vi "svc_Complex to Mag2 Spectrum.vi"(4 "complex spectrum":cluster{"f0":dbl, "df":dbl, "spectrum":cdb[]} {"spectrum" format="%.2f"; "df" format="%.2f"; "f0" format="%.2f"}) -> (1 "power spectrum":cluster{"f0":dbl, "df":dbl, "spectrum":dbl[]} {"spectrum" format="%.2f"; "df" format="%.2f"; "f0" format="%.2f"})   [LabVIEW 2017]
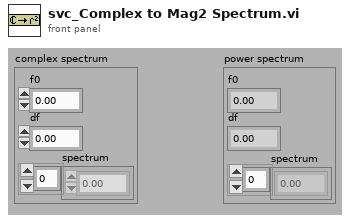
[diagram p1: front panel]
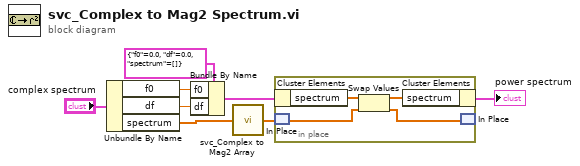
[diagram p0: block diagram]
diagram:
  n1 = Unbundle By Name("complex spectrum") -> ("f0"=w6:dbl, "df"=w7:dbl, "spectrum"=w5:cdb[])
  n2 = Bundle By Name(cluster=cluster{"f0":dbl, "df":dbl, "spectrum":dbl[]} {"f0"=0.0, "df"=0.0, "spectrum"=[]} ("power spectrum"), "f0"=w6, "df"=w7) -> (w2:cluster{"f0":dbl, "df":dbl, "spectrum":dbl[]})
  n3 = call <vilib>:"svc_Complex to Mag2 Array.vi"("complex array"=w5) -> ("magnitude^2 array"=w3:dbl[])  [unwired: 4 in]
  n4 = in-place {
    n5 = in-place-cluster #1(w2) -> ("spectrum"=w12:dbl[])
    n6 = in-place-match #2(w3) -> (w10:dbl[])
    n7 = Swap Values(12:w12, 14:w10) -> (1:w11:dbl[], 3:w9:dbl[])  [unwired: 1 in]
    n8 = in-place-cluster #1("spectrum"=w11) -> (→"power spectrum":cluster{"f0":dbl, "df":dbl, "spectrum":dbl[]})
    n9 = in-place-match #2(w9) -> ()  [unwired: 1 out]
  }
